vi "p5.vi"() -> ()   [LabVIEW 2015]
panel:
  out "x = y?":bool
  out "Array 2":i32[](array[numeric])
  out "N 2":i32
  out "i 2":i32
  out "Add":i32
  out "i":i32
  out "N":i32
  out "Array":i32[](array[numeric])
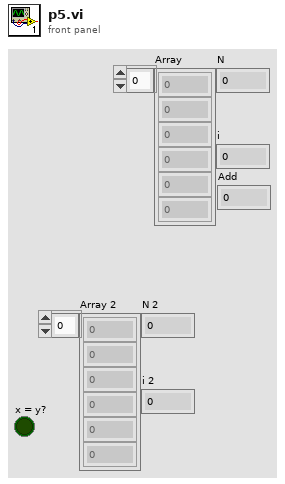
[diagram p1: front panel]
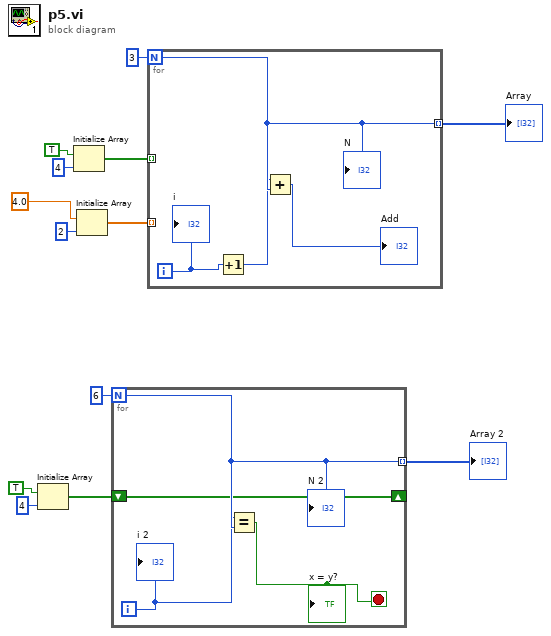
[diagram p0: block diagram]
diagram:
  n1 = Initialize Array(TRUE, 4 ("dimension size")) -> (w4:bool[])
  n2 = Initialize Array(TRUE, 4 ("dimension size")) -> (w12:bool[])
  n3 = Initialize Array(4.0 ("dimension size"), 2 ("dimension size")) -> (w6:dbl[])
  n4 = for {
    N: 6 -> [w17]
    tunnel: [w17] -> w1 mode=indexing
    shift-right: [w14] -> _
    shift-left: w4 -> [w14]
    i -> [w16]
    stop <- w15 stop-if-true
    n5 = Equal?(x=w16, y=w17) -> (x = y?=w15:bool)
    "x = y?" <- w15
    "N 2" <- w17
    "i 2" <- w16
  }
  "Array 2" <- w1
  n6 = for {
    N: 3 -> [w21]
    tunnel: w12 -> [_] mode=indexing
    tunnel: [w21] -> w9 mode=indexing
    tunnel: w6 -> [_] mode=indexing
    i -> [w20]
    n7 = Increment(x=w20) -> (x+1=w19:i32)
    n8 = Add(x=w19, y=w21) -> (x+y=→"Add":i32)
    "N" <- w21
    "i" <- w20
  }
  "Array" <- w9
